vi "Ryan click here.vi"   [LabVIEW 2016]
types:
  T1 = typedef "LVHSConnector.ctl" = refnum<class "BrickReference.lvclass">
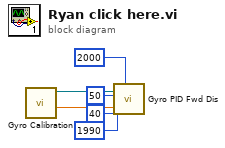
[diagram p0: block diagram]
diagram:
  n1 = call "Gyro Calibration.vi"() -> ("Degrees"=w6:sgl, "NXT/EV3"=w4:T1)  [unwired: 7 in, 1 out]
  n2 = call "Gyro PID Fwd Dis.vi"("Target angle"=w6, "Threshold to stop"=2000, "Threshold to slow"=1990, "Min. speed"=40, "Max. speed"=50, "EV3 in"=w4) -> ()  [unwired: 5 in, 1 out]
